vi "Test Execute SQL Query (blob as I32).vi"(8 "error in (no error)":errorcluster, 10 "query":string="SELECT * from blobs;", 11 "database in":path=path "C:/labview/sqlite_dbManager/test database/blob.db") -> (0 "error out":errorcluster, 1 "Query Result":string[][](array[string]), 2 "nonzero result?":bool)   [LabVIEW 2020, in "sqlite3.lvlib"]
uses:
  sqlite3.lvlib
  sqlite/VIs/open v2.vi
  sqlite/VIs/prepare v2.vi
  sqlite/VIs/step.vi
  sqlite/VIs/column count.vi
  compound/Column.vi
  compound/Resolve Result Type.vi
  sqlite/VIs/finalize.vi
  sqlite/VIs/close v2.vi
  sqlite/subvi/Error Converter (ErrCode or Status).vi
  sqlite/VIs/column text.vi
  sqlite/VIs/column bytes.vi
  sqlite/VIs/column blob.vi
  utilities/MoveBlock.vi
  sqlite/VIs/column type.vi
  sqlite/VIs/errstr.vi
panel:
  out "Pictures":picture[](array[picture])
  # "can only read columns as blobs if they are created \nas blobs.  trying to read another column affinity as a blob won't work"
  # "In general, blobs are good when under 100kb.  \nif larger, store the file name and keep it externally."
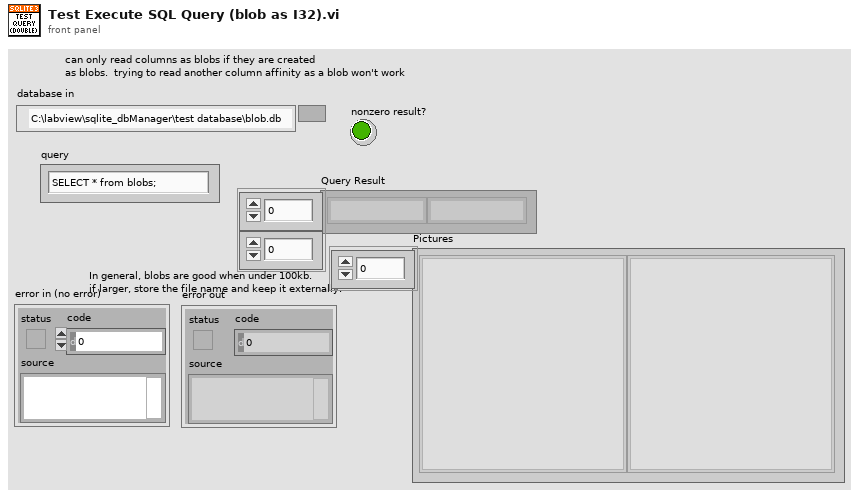
[diagram p1: front panel]
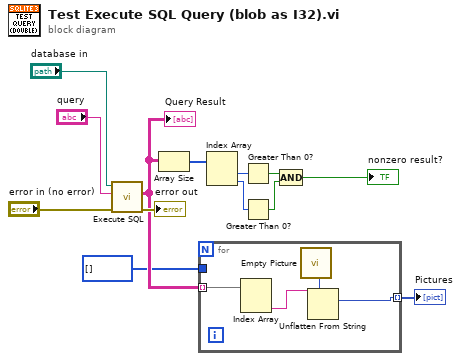
[diagram p0: block diagram]
diagram:
  n1 = call "Execute SQL.vi"("error in (no error)"="error in (no error)", "sql (string)"="query", "database in"="database in") -> ("error out"=→"error out":errorcluster, "Query Result"=w2:string[][])  [unwired: 7 in]
  "Query Result" <- w2
  n2 = Array Size(array=w2) -> (size(s)=w9:i32[])
  n3 = for {
    tunnel: w2 -> [w15] mode=indexing
    tunnel: [w16] -> w3 mode=indexing
    tunnel: u8[] [] -> [_]
    n4 = Index Array(array=w15) -> (element #2=w14:string)  [unwired: 2 in, 1 out]
    n5 = call "Empty Picture"() -> ("empty picture"=w17:picture)
    n6 = Unflatten From String(type=w17, binary string=w14) -> (value=w16:picture)  [unwired: 3 in, 2 out]
  }
  "Pictures" <- w3
  n7 = Index Array(array=w9) -> (element #1=w8:i32, element #2=w7:i32)  [unwired: 2 in]
  n8 = Greater Than 0?(x=w8) -> (x > 0?=w6:bool)
  n9 = Greater Than 0?(x=w7) -> (x > 0?=w5:bool)
  n10 = Compound Arithmetic op=AND(w6, w5) -> (→"nonzero result?":bool)
